vi "Raster_Scan_FSRS.vi"() -> ()   [LabVIEW 2014] (continued)
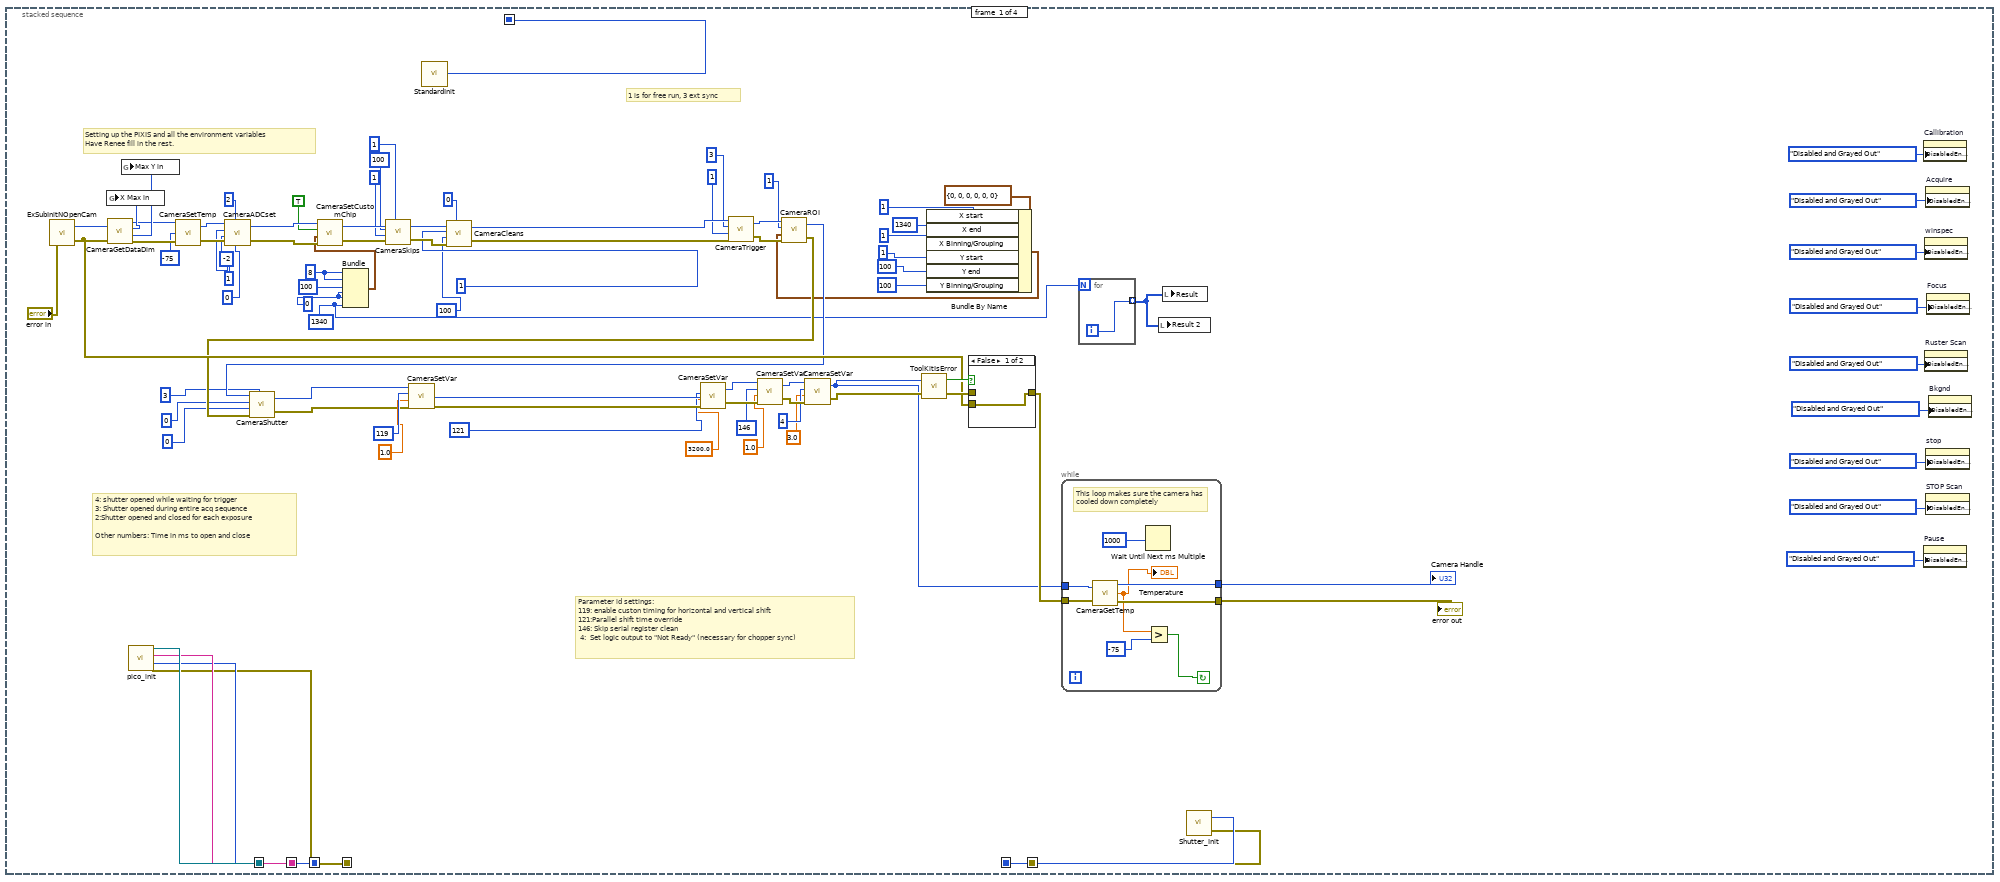
[diagram p2: hidden frame]
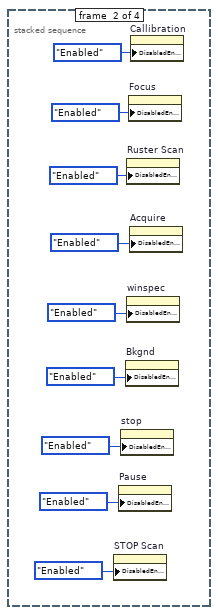
[diagram p4: hidden frame]
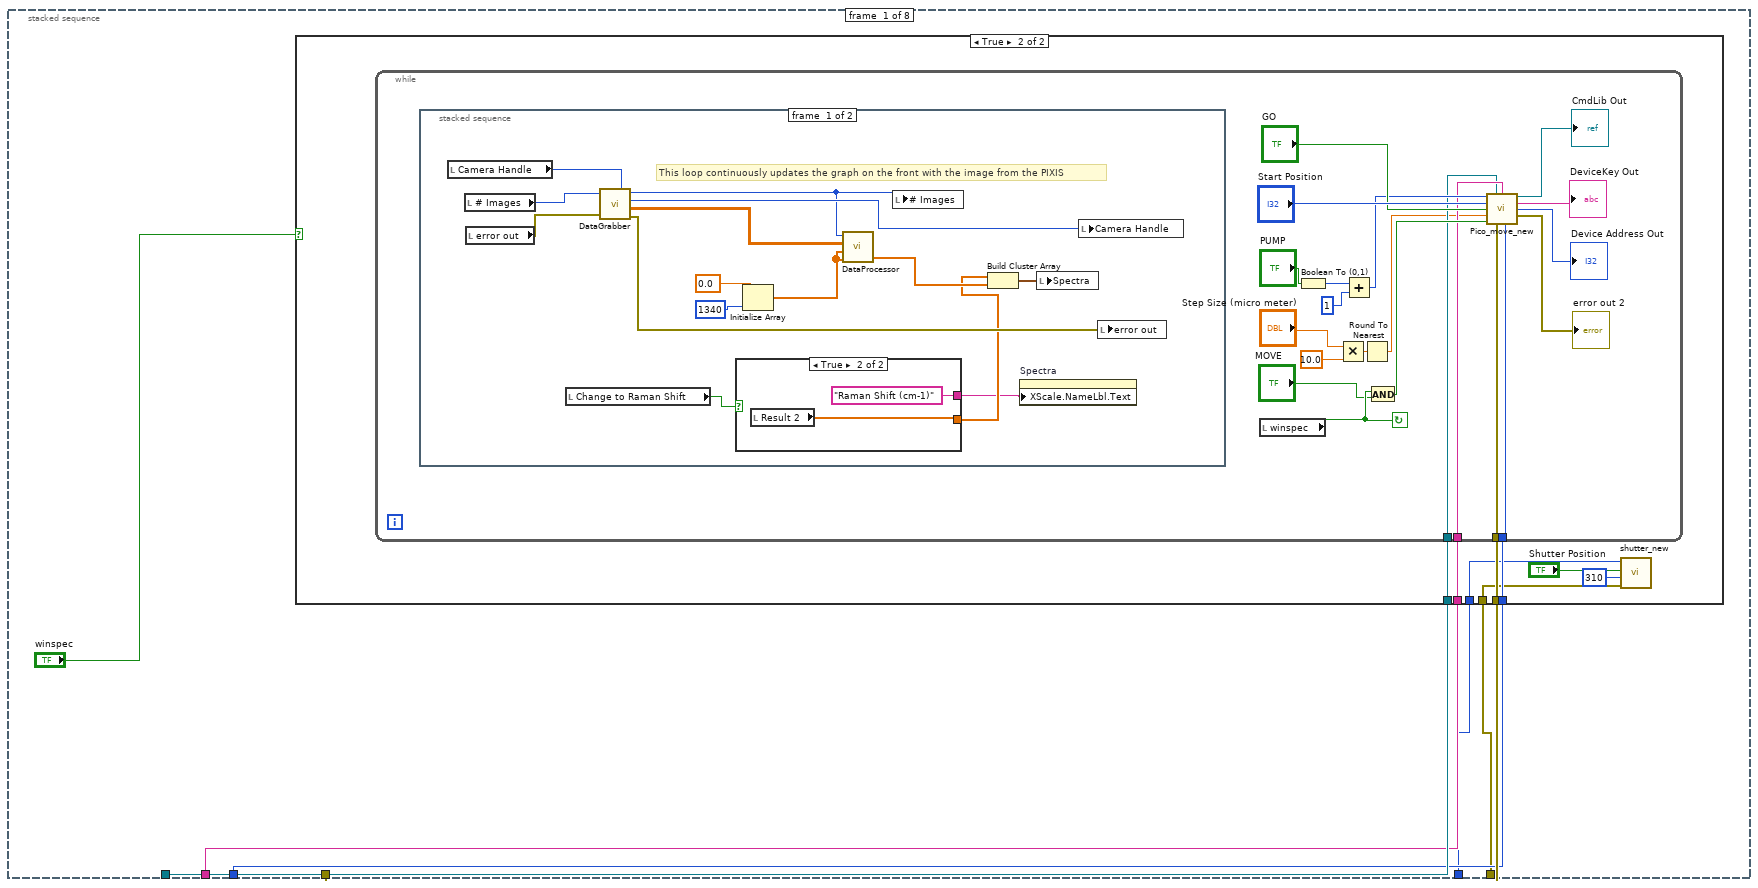
[diagram p5: hidden frame]
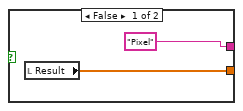
[diagram p7: hidden frame]
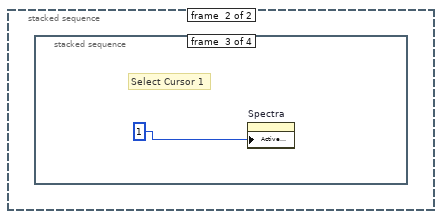
[diagram p8: hidden frame]
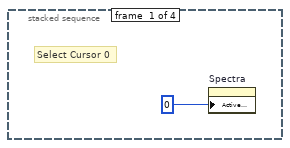
[diagram p9: hidden frame]
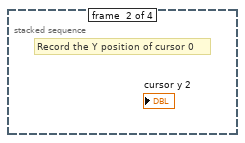
[diagram p10: hidden frame]
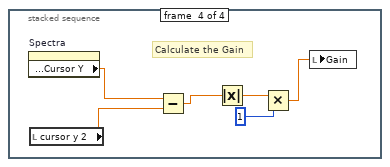
[diagram p11: hidden frame]
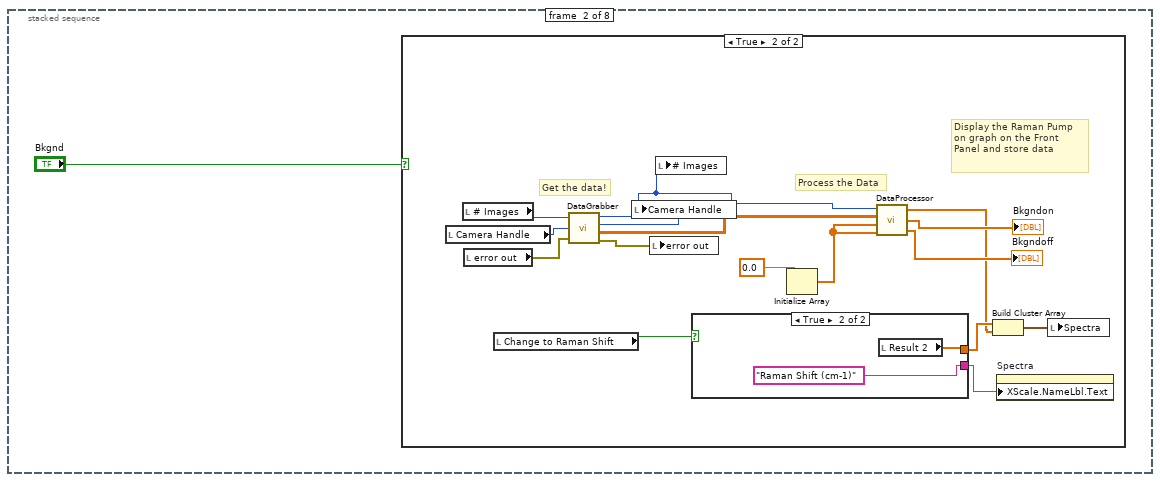
[diagram p12: hidden frame]
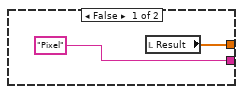
[diagram p14: hidden frame]
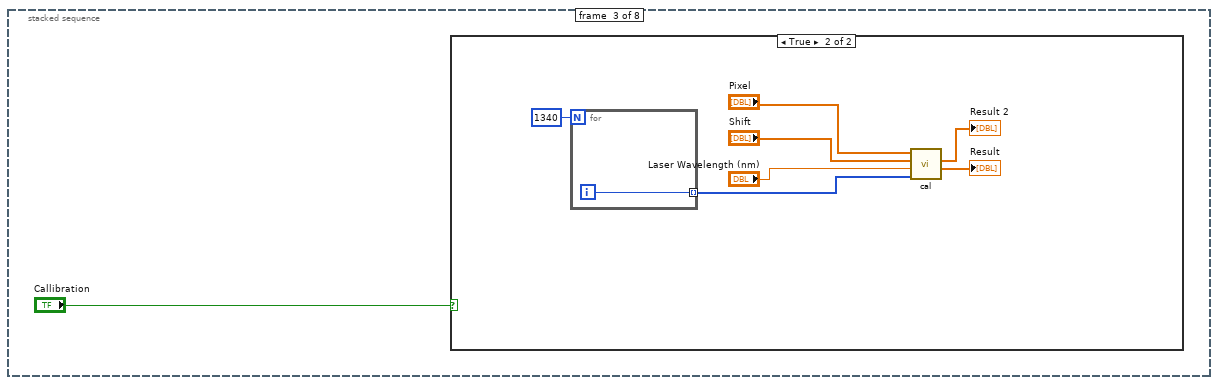
[diagram p15: hidden frame]
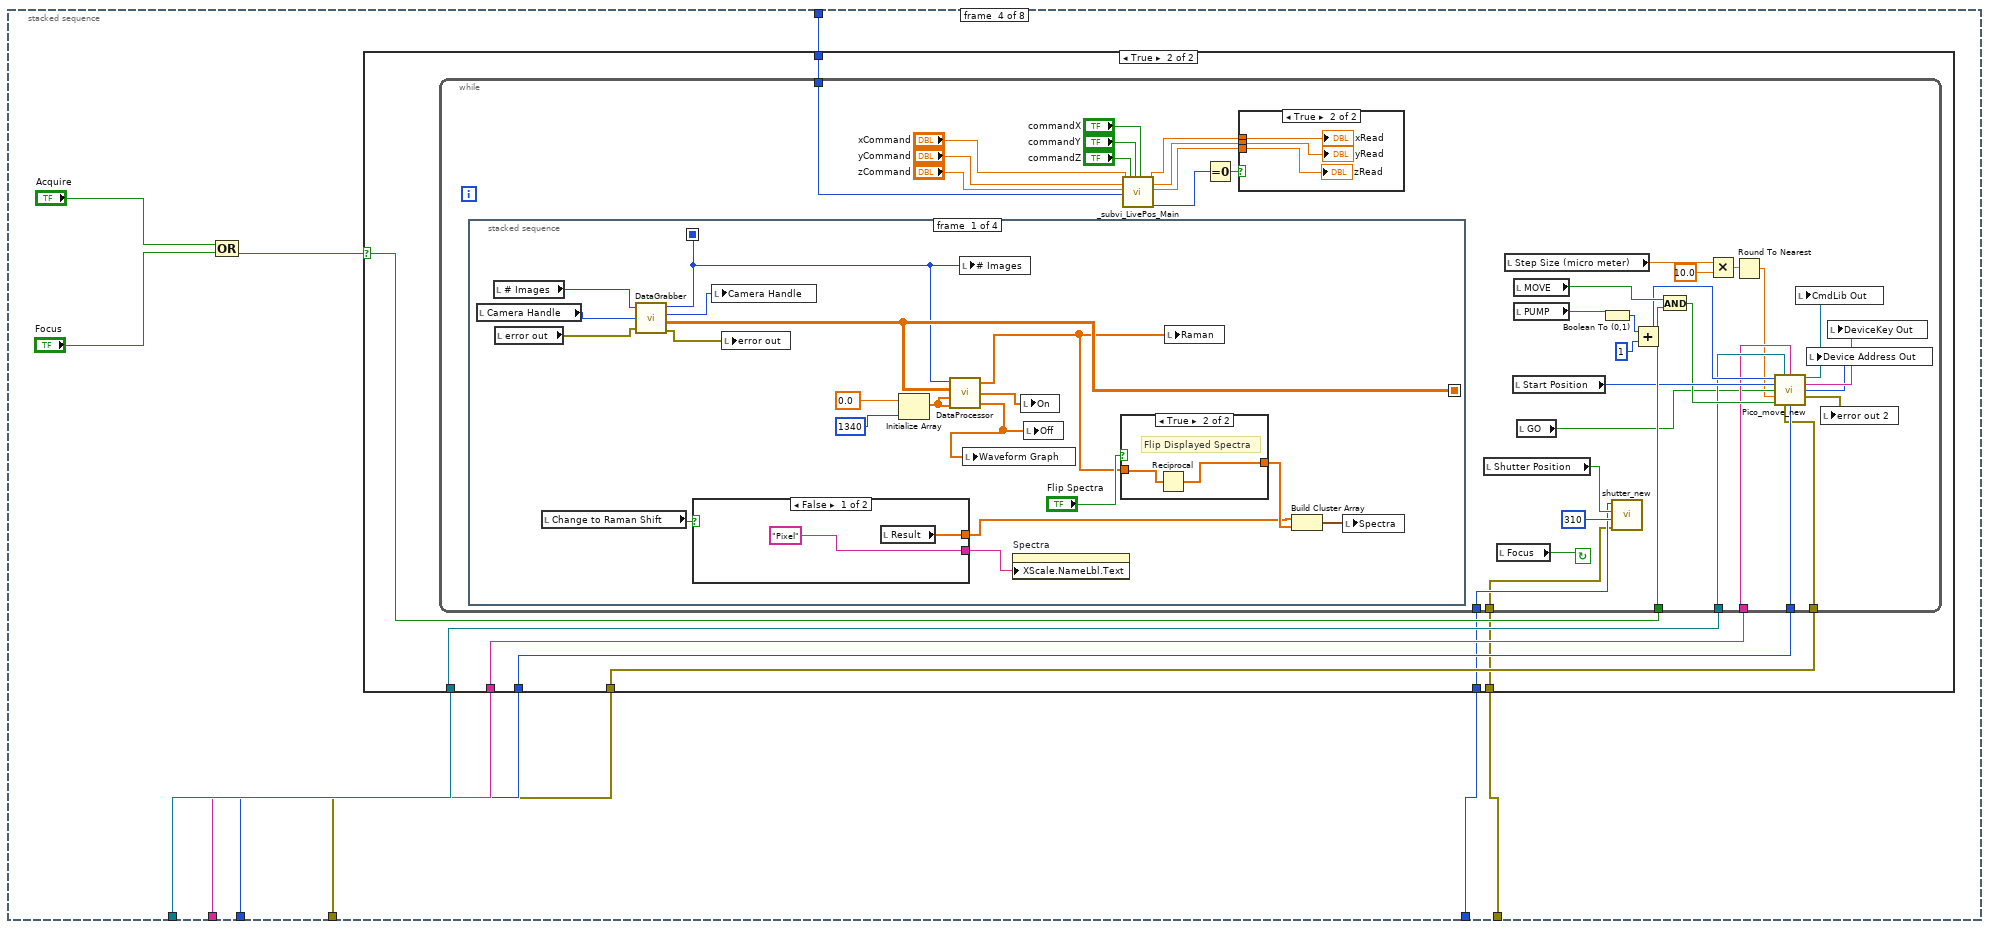
[diagram p17: hidden frame]
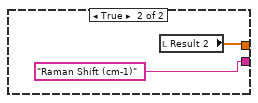
[diagram p20: hidden frame]
                      n390 = Array Size(array="Timepoints") -> (size(s)=w773:i32)
                      n391 = for {
                        N: w773 -> [_]
                        tunnel: "Timepoints" -> [w776]
                        tunnel: w770 -> [w775]
                        tunnel: w771 -> [_]
                        tunnel: w770 -> [_]
                        i -> [w774]
                        n392 = stacked-sequence {
                          seq-local: [_ _ _ w847 _ _ _ _ _ _] -> [_ _ _ _ _ w863 _ _ _ _]
                          seq-local: [_ _ _ w845 _ _ _ _ _ _] -> [_ _ _ _ _ w860 _ _ _ _]
                          tunnel: w774 -> [w778 w828 _ _ _ _ w872 _ _ _]
                          tunnel: w776 -> [_ w829 _ _ _ _ w871 _ _ _]
                          tunnel: w775 -> [w780 _ _ _ _ _ w869 _ _ _]
                          frame #0 {
                            n393 = local read "GndNum"() -> (w779:u32)
                            n394 = Quotient & Remainder(x=w778, y=w779) -> (x-y*floor(x/y)=w782:u32, floor(x/y)=w777:u32)
                            n395 = Equal To 0?(x=w782) -> (x = 0?=w781:bool)
                            n396 = case shown="True" w781 {
                              tunnel: w780 -> [_ w784]
                              tunnel: w777 -> [_ w783]
                              frame False {
                              }
                              frame True {
                                # "Here we take a ground spectrum"
                                n397 = stacked-sequence {
                                seq-local: [w795 _] -> [_ _]
                                tunnel: w784 -> [_ w818]
                                tunnel: w783 -> [_ w808]
                                frame #0 {
                                n398 = local read "Camera Handle 2"() -> (w801:u32)
                                n399 = local read "# Images 2"() -> (w795:u16)
                                n400 = local read "error out 3"() -> (w800:errorcluster)
                                n401 = call "DataGrabber.vi"("# Images In"=w795, "Camera Handle"=w801, "error in (no error)"=w800) -> ("# Images Out"=w790:u16, "Camera Handle"=w798:u32, "Data"=w796:dbl[][], "error out"=w799:errorcluster)
                                n402 = local write "Camera Handle 2"(w798) -> ()
                                n403 = local write "error out 3"(w799) -> ()
                                n404 = local write "# Images 2"(w790) -> ()
                                n405 = local read "Change to Raman Shift 2"() -> (w786:bool)
                                n406 = local read "Bkgndoff 2"() -> (w793:dbl[])
                                n407 = local read "Bkgndon 2"() -> (w794:dbl[])
                                n408 = local read "Flip Spectra 2"() -> (w797:bool)
                                n409 = call "DataProcessor.vi"("PumpOffBkgd"=w793, "PumpOnBkgd"=w794, "Data"=w796, "# of Images"=w790) -> ("PumpOff"=w785:dbl[], "PumpOn"=w791:dbl[], "Raman"=w792:dbl[])
                                "Ground 2" <- w792
                                n410 = local write "Wave"(w785) -> ()
                                n411 = local write "On"(w791) -> ()
                                n412 = local write "Off"(w785) -> ()
                                n413 = case shown="False" w786 {
                                tunnel: [w802 w803] -> w787
                                frame False {
                                n414 = local read "Result 4"() -> (w802:dbl[])
                                }
                                frame True {
                                n415 = local read "Result 3"() -> (w803:dbl[])
                                }
                                }
                                n416 = case shown="True" w797 {
                                tunnel: w792 -> [w804 w806]
                                tunnel: [w804 w805] -> w789
                                frame False {
                                }
                                frame True {
                                n417 = Reciprocal(x=w806) -> (1/x=w805:dbl[])
                                }
                                }
                                n418 = Build Cluster Array(w787, w789) -> (w788:cluster{dbl, dbl}[])
                                n419 = local write "Spectra"(w788) -> ()
                                }
                                frame #1 {
                                # "Here we save the ground spectrum"
                                n420 = local read "Filename 2"() -> (w820:string)
                                n421 = local read "Path 2"() -> (w822:string)
                                n422 = Format Into String(w818) -> (resulting string=w817:string)  [unwired: 3 in, 1 out]
                                n423 = Format Into String(w808) -> (resulting string=w810:string)  [unwired: 3 in, 1 out]
                                n424 = Concatenate Strings(w822, "\\", w820, "_", w817, "_", w810, "gr") -> (w816:string)
                                n425 = local read "Ground"() -> (w807:dbl[])
                                n426 = local read "On"() -> (w824:dbl[])
                                n427 = local read "Off"() -> (w823:dbl[])
                                n428 = String To Path(string=w816) -> (path=w812:path)
                                n429 = Build Array(w807, w824, w823) -> (w813:dbl[][])
                                n430 = call-poly <vilib>:"Write To Spreadsheet File.vi"("transpose? (no:F)"=TRUE, "format (%.3f)"="%.7f", "2D data"=w813, "file path (dialog if empty)"=w812) -> ()  [unwired: 4 in, 1 out]
                                }
                                }
                              }
                            }
                          }
                          frame #1 {
                            n431 = Index Array(array=w829, index=w828) -> (element=w827:dbl)
                            n432 = local read "t=0 Position"() -> (w831:dbl)
                            n433 = Multiply(x=w827, y=0.00015) -> (x*y=w834:dbl)
                            n434 = Add(x=w834, y=w831) -> (x+y=w826:dbl)
                            n435 = Absolute Value(x=w826) -> (abs(x)=w833:dbl)
                            n436 = Less?(x=w833, y=49.9) -> (x < y?=w825:bool)
                            n437 = case shown="True" w825 {
                              tunnel: w826 -> [_ w838]
                              frame False {
                              }
                              frame True {
                                n438 = local read "PI Stage Error"() -> (w837:errorcluster)
                                n439 = call "pi_scan.vi"("error in"=w837, "Start Position"=w838) -> ("error out"=w836:errorcluster, "element"=w835:dbl)  [unwired: 8 in]
                                n440 = Build Array(w835) -> (w839:dbl[])
                                n441 = local write "PI Stage Error"(w836) -> ()
                                n442 = local write "Position"(w839) -> ()
                              }
                            }
                          }
                          frame #2 {
                            # "Open Actinic Pump shutter"
                            n443 = call "shutter.vi"("error in"="shutter error in", "Shutter Position"=TRUE) -> ("error out"=→"shutter error out":errorcluster, "Status"=→"Shutter status":string)  [unwired: 1 in]
                            n444 = Wait (ms)(milliseconds to wait=50) -> ()  [unwired: 1 out]
                          }
                          frame #3 {
                            # "Here we take the data for the given time point"
                            n445 = local read "Camera Handle 2"() -> (w850:u32)
                            n446 = local read "error out 3"() -> (w851:errorcluster)
                            n447 = call "DataGrabber.vi"("# Images In"="# Images 2", "Camera Handle"=w850, "error in (no error)"=w851) -> ("# Images Out"=w845:u16, "Camera Handle"=w848:u32, "Data"=w847:dbl[][], "error out"=w846:errorcluster)
                            n448 = local write "Camera Handle 2"(w848) -> ()
                            n449 = local write "error out 3"(w846) -> ()
                            n450 = local write "# Images 2"(w845) -> ()
                          }
                          frame #4 {
                            # "Actinic Pump Shutter Close"
                            n451 = local read "shutter error in"() -> (w855:errorcluster)
                            n452 = call "shutter.vi"("error in"=w855, "Shutter Position"=FALSE) -> ("error out"=w853:errorcluster, "Status"=w854:string)  [unwired: 1 in]
                            n453 = local write "shutter error out"(w853) -> ()
                            n454 = local write "Shutter status"(w854) -> ()
                            n455 = Wait (ms)(milliseconds to wait=50) -> ()  [unwired: 1 out]
                          }
                          frame #5 {
                            n456 = local read "Bkgndon 2"() -> (w862:dbl[])
                            n457 = local read "Bkgndoff 2"() -> (w861:dbl[])
                            n458 = call "DataProcessor.vi"("PumpOffBkgd"=w861, "PumpOnBkgd"=w862, "Data"=w863, "# of Images"=w860) -> ("PumpOff"=w857:dbl[], "PumpOn"=→"On 2":dbl[], "Raman"=→"Raman 2":dbl[])
                            n459 = local write "Wave"(w857) -> ()
                          }
                          frame #6 {
                            n460 = Index Array(array=w871, index=w872) -> (element=w870:dbl)
                            n461 = call "tppathcr.vi"("input"=w870) -> ("out"=w873:string)
                            n462 = Format Into String(w869) -> (resulting string=w868:string)  [unwired: 3 in, 1 out]
                            n463 = Concatenate Strings("Path 2", "\\", "Filename 2", "_", w873, "exc", w868) -> (w879:string)
                            n464 = local read "Raman 2"() -> (w864:dbl[])
                            n465 = local read "On 2"() -> (w867:dbl[])
                            n466 = local read "Off"() -> (w866:dbl[])
                            n467 = String To Path(string=w879) -> (path=w875:path)
                            n468 = Build Array(w864, w867, w866) -> (w880:dbl[][])
                            n469 = call-poly <vilib>:"Write To Spreadsheet File.vi"("transpose? (no:F)"=TRUE, "format (%.3f)"="%.7f", "2D data"=w880, "file path (dialog if empty)"=w875) -> ()  [unwired: 4 in, 1 out]
                          }
                          frame #7 {
                            n470 = case shown="True" "ShowRaw" {
                              frame False {
                                n471 = local read "Flip Spectra 2"() -> (w892:bool)
                                n472 = local read "Ground 2"() -> (w890:dbl[])
                                n473 = local read "Raman 2"() -> (w891:dbl[])
                                n474 = local read "Change to Raman Shift 2"() -> (w884:bool)
                                n475 = case shown="True" w892 {
                                tunnel: w891 -> [w896 w900]
                                tunnel: [w896 w899] -> w889
                                tunnel: w890 -> [w895 w898]
                                tunnel: [w895 w897] -> w888
                                frame False {
                                }
                                frame True {
                                n476 = Reciprocal(x=w898) -> (1/x=w897:dbl[])
                                n477 = Reciprocal(x=w900) -> (1/x=w899:dbl[])
                                }
                                }
                                n478 = case shown="True" w884 {
                                tunnel: [w893 w894] -> w885
                                frame False {
                                n479 = local read "Result 3"() -> (w893:dbl[])
                                }
                                frame True {
                                n480 = local read "Result 4"() -> (w894:dbl[])
                                }
                                }
                                n481 = Subtract(x=w889, y=w888) -> (x-y=w887:dbl[])
                                n482 = Build Cluster Array(w885, w887) -> (w886:cluster{dbl, "Numeric":dbl}[])
                                n483 = local write "Spectra"(w886) -> ()
                              }
                              frame True {
                                n484 = local read "Flip Spectra 2"() -> (w905:bool)
                                n485 = local read "Change to Raman Shift 2"() -> (w902:bool)
                                n486 = local read "Raman 2"() -> (w906:dbl[])
                                n487 = case shown="False" w905 {
                                tunnel: w906 -> [w909 w911]
                                tunnel: [w909 w910] -> w904
                                frame False {
                                }
                                frame True {
                                n488 = Reciprocal(x=w911) -> (1/x=w910:dbl[])
                                }
                                }
                                n489 = case shown="True" w902 {
                                tunnel: [w907 w908] -> w903
                                frame False {
                                n490 = local read "Result 3"() -> (w907:dbl[])
                                }
                                frame True {
                                n491 = local read "Result 4"() -> (w908:dbl[])
                                }
                                }
                                n492 = Build Cluster Array(w903, w904) -> (w901:cluster{dbl, "Numeric":dbl}[])
                                n493 = local write "Spectra"(w901) -> ()
                              }
                            }
                          }
                          frame #8 {
                            n494 = stacked-sequence {
                              frame #0 {
                                n495 = property on="Spectra" class="XYGraph (strict)"("Active Cursor"=0) -> ()  [unwired: 2 in, 2 out]
                              }
                              frame #1 {
                                n496 = property on="Spectra" class="XYGraph (strict)"() -> ("Cursor.Cursor Position:Cursor Y"=w914:dbl)  [unwired: 2 in, 2 out]
                                n497 = local read "Change to Raman Shift 2"() -> (w915:bool)
                                n498 = local write "cursor y"(w914) -> ()
                                n499 = case shown="False" w915 {
                                tunnel: ["Pixel" ("X Scale.Name Label.Text") "Raman Shift (cm-1)" ("X Scale.Name Label.Text")] -> w913
                                frame False {
                                }
                                frame True {
                                }
                                }
                                n500 = property on="Spectra" class="XYGraph (strict)"("XScale.NameLbl.Text"=w913) -> ()  [unwired: 2 in, 2 out]
                              }
                              frame #2 {
                                n501 = property on="Spectra" class="XYGraph (strict)"("Active Cursor"=1) -> ()  [unwired: 2 in, 2 out]
                              }
                              frame #3 {
                                n502 = property on="Spectra" class="XYGraph (strict)"() -> ("Cursor.Cursor Position:Cursor Y"=w919:dbl)  [unwired: 2 in, 2 out]
                                n503 = local read "cursor y"() -> (w920:dbl)
                                n504 = Subtract(x=w919, y=w920) -> (x-y=w922:dbl)
                                n505 = Absolute Value(x=w922) -> (abs(x)=w924:dbl)
                                n506 = Multiply(x=w924, y=100) -> (x*y=w921:dbl)
                                n507 = local write "Gain 2"(w921) -> ()
                              }
                            }
                          }
                          frame #9 {
                            n508 = while {
                              stop <- "Pause 2" continue-if-true
                            }
                          }
                        }
                      }
                    }
                  }
                }
              }
            }
          }
          frame #6 {
            n509 = case shown="True" "Save" {
              frame False {
              }
              frame True {
                n510 = local read "Raman"() -> (w949:dbl[])
                n511 = local read "Off"() -> (w947:dbl[])
                n512 = local read "On"() -> (w948:dbl[])
                n513 = local read "Path"() -> (w946:string)
                n514 = Build Array(w949, w948, w947) -> (w940:dbl[][])
                n515 = local read "Filename"() -> (w944:string)
                n516 = Concatenate Strings(w946, "\\", w944) -> (w943:string)
                n517 = String To Path(string=w943) -> (path=w939:path)
                n518 = call-poly <vilib>:"Write To Spreadsheet File.vi"("transpose? (no:F)"=TRUE, "format (%.3f)"="%.7f", "2D data"=w940, "file path (dialog if empty)"=w939) -> ()  [unwired: 4 in, 1 out]
              }
            }
            n519 = case shown="True" "subtract" {
              frame False {
              }
              frame True {
                n520 = local read "Change to Raman Shift"() -> (w957:bool)
                n521 = local read "Subtrarray"() -> (w961:dbl[])
                n522 = local read "Raman"() -> (w960:dbl[])
                n523 = Multiply(x="Scale factor", y=w961) -> (x*y=w959:dbl[])
                n524 = Subtract(x=w960, y=w959) -> (x-y=w955:dbl[])
                n525 = case shown="True" w957 {
                  tunnel: [w964 w966] -> w956
                  tunnel: ["Pixel" ("X Scale.Name Label.Text") "Raman Shift (cm-1)" ("X Scale.Name Label.Text")] -> w958
                  frame False {
                    n526 = local read "Result"() -> (w964:dbl[])
                  }
                  frame True {
                    n527 = local read "Result 2"() -> (w966:dbl[])
                  }
                }
                n528 = property on="Spectra" class="XYGraph (strict)"("XScale.NameLbl.Text"=w958) -> ()  [unwired: 2 in, 2 out]
                n529 = Build Cluster Array(w956, w955) -> (w954:cluster{dbl, dbl}[])
                n530 = local write "Spectra"(w954) -> ()
              }
            }
            n531 = case shown="True" "ChooseBkgdFile" {
              frame False {
              }
              frame True {
                n532 = call-poly <vilib>:"Read From Spreadsheet File.vi"("transpose (no:F)"=TRUE) -> ("first row"=w968:dbl[], "new file path (Not A Path if cancelled)"=→"Background File":path)  [unwired: 6 in, 3 out]
                n533 = Array Subset(array=w968, index=0, length=1340) -> (→"Subtrarray":dbl[])
              }
            }
            n534 = case shown="True" "SetPath" {
              frame False {
              }
              frame True {
                (unwired) 5
                n535 = File Dialog(11:path "C:/DATA") -> (0:w950:errorcluster, 3:w953:path)  [unwired: 6 in, 2 out]
                n536 = Unbundle(w950) -> ()  [unwired: 3 out]
                n537 = Path To String(path=w953) -> (string=w951:string)
                n538 = local write "Path"(w951) -> ()
              }
            }
            n539 = case shown="True" "Boolean" {
              frame False {
              }
              frame True {
                n540 = local read "Path"() -> (w935:string)
                n541 = local read "Filename"() -> (w937:string)
                n542 = Concatenate Strings(w935, "\\", w937) -> (w938:string)
                n543 = String To Path(string=w938) -> (path=w934:path)
                n544 = local read "Off"() -> (w931:dbl[])
                n545 = call-poly <vilib>:"Write To Spreadsheet File.vi"("transpose? (no:F)"=TRUE, "format (%.3f)"="%.7f", "1D data"=w931, "file path (dialog if empty)"=w934) -> ()  [unwired: 4 in, 1 out]
              }
            }
          }
          frame #7 {
            n546 = case shown="True" "Time" {
              frame False {
              }
              frame True {
                n547 = while {
                  shift-right: [w975] -> _
                  shift-left: _ -> [w974]
                  i -> [w976]
                  stop <- "?" stop-if-true
                  n548 = stacked-sequence {
                    seq-local: [w978 _ _] -> [_ _ w1024]
                    tunnel: w976 -> [_ w1005 _]
                    tunnel: [_ _ w1021] -> w975
                    tunnel: w974 -> [_ _ w1020]
                    frame #0 {
                      n549 = local read "Change to Raman Shift"() -> (w980:bool)
                      n550 = local read "# Images"() -> (w979:u16)
                      n551 = local read "Camera Handle"() -> (w996:u32)
                      n552 = local read "error out"() -> (w995:errorcluster)
                      n553 = call "DataGrabber.vi"("# Images In"=w979, "Camera Handle"=w996, "error in (no error)"=w995) -> ("# Images Out"=w989:u16, "Camera Handle"=w993:u32, "Data"=w992:dbl[][], "error out"=w994:errorcluster)
                      n554 = local write "Camera Handle"(w993) -> ()
                      n555 = local write "error out"(w994) -> ()
                      n556 = case shown="False" w980 {
                        tunnel: [w998 w1000] -> w978
                        tunnel: ["Pixel" ("X Scale.Name Label.Text") "Raman Shift (cm-1)" ("X Scale.Name Label.Text")] -> w982
                        frame False {
                          n557 = local read "Result"() -> (w998:dbl[])
                        }
                        frame True {
                          n558 = local read "Result 2"() -> (w1000:dbl[])
                        }
                      }
                      n559 = local write "# Images"(w989) -> ()
                      n560 = local read "Bkgndoff"() -> (w990:dbl[])
                      n561 = local read "Bkgndoff"() -> (w991:dbl[])
                      n562 = call "DataProcessor.vi"("PumpOffBkgd"=w990, "PumpOnBkgd"=w991, "Data"=w992, "# of Images"=w989) -> ("PumpOff"=w988:dbl[], "PumpOn"=w987:dbl[], "Raman"=w981:dbl[])
                      n563 = local read "Flip Spectra"() -> (w984:bool)
                      n564 = property on="Spectra" class="XYGraph (strict)"("XScale.NameLbl.Text"=w982) -> ()  [unwired: 2 in, 2 out]
                      n565 = local write "On"(w987) -> ()
                      n566 = local write "Off"(w988) -> ()
                      n567 = Not(x=w984) -> (.not. x?=w985:bool)
                      n568 = case shown="True" w985 {
                        tunnel: w981 -> [w1001 w1003]
                        tunnel: [w1002 w1003] -> w986
                        frame False {
                          n569 = Reciprocal(x=w1001) -> (1/x=w1002:dbl[])
                        }
                        frame True {
                        }
                      }
                      n570 = Build Cluster Array(w978, w986) -> (w983:cluster{dbl, dbl}[])
                      n571 = local write "Spectra"(w983) -> ()
                      n572 = local write "Raman"(w981) -> ()
                    }
                    frame #1 {
                      # "Here we save spectrum for each special point"
                      n573 = Increment(x=w1005) -> (x+1=w1004:i32)
                      n574 = local read "Filename"() -> (w1008:string)
                      n575 = local read "Path"() -> (w1010:string)
                      n576 = Format Into String(w1004) -> (resulting string=w1006:string)  [unwired: 3 in, 1 out]
                      n577 = Concatenate Strings(w1010, "\\", w1008, "_", w1006) -> (w1011:string)
                      n578 = local read "Off"() -> (w1018:dbl[])
                      n579 = local read "On"() -> (w1017:dbl[])
                      n580 = local read "Raman"() -> (w1014:dbl[])
                      n581 = String To Path(string=w1011) -> (path=w1015:path)
                      n582 = Build Array(w1014, w1018, w1017) -> (w1016:dbl[][])
                      n583 = local write "File_name"(w1011) -> ()
                      n584 = call-poly <vilib>:"Write To Spreadsheet File.vi"("transpose? (no:F)"=TRUE, "format (%.3f)"="%.7f", "2D data"=w1016, "file path (dialog if empty)"=w1015) -> ()  [unwired: 4 in, 1 out]
                    }
                    frame #2 {
                      # "Peak fitting and intergation"
                      n585 = local read "Raman"() -> (w1025:dbl[])
                      n586 = property on="Spectra" class="XYGraph (strict)"("Active Cursor"=u32 1) -> ("Cursor.Cursor X"=w1027:dbl)  [unwired: 2 in, 2 out]
                      n587 = local read "Enum"() -> (w1022:enum16{"Lorantzian", "fano", "gaussian"})
                      n588 = property on="Spectra" class="XYGraph (strict)"("Active Cursor"=u32 0) -> ("Cursor.Cursor X"=w1028:dbl)  [unwired: 2 in, 2 out]
                      n589 = call "fit_new.vi"("Cursor1 2"=w1027, "Cursor1"=w1028, "array 2"=w1024, "array"=w1025, "Enum"=w1022, "Initial Parameters"="Fano initial Parameters 2") -> ("Intergrate"=w1023:dbl, "Fit"=w1019:dbl)  [unwired: 4 in]
                      n590 = local write "FIT"(w1019) -> ()
                      n591 = local write "AREA"(w1023) -> ()
                      n592 = Build Array (concatenate)(w1020, w1019) -> (w1021:dbl[])
                      "Waveform Graph" <- w1021
                    }
                  }
                }
              }
            }
          }
        }
      }
    }
    frame #3 {
      n593 = local read "DeviceKey Out"() -> (w1033:string)
      n594 = local read "error out 2"() -> (w1032:errorcluster)
      n595 = local read "CmdLib Out"() -> (w1034:refnum<k24>)
      n596 = stacked-sequence {
        frame #0 {
          n597 = local read "Camera Handle"() -> (w1035:u32)
          n598 = local read "error out"() -> (w1036:errorcluster)
          n599 = call <userlib>:"CameraClose.vi"("error in"=w1036, "Camera Handle"=w1035) -> ("error out"=w1038:errorcluster)
          n600 = call <userlib>:"UninitToolkit.vi"("error in"=w1038) -> ("error out"=w1037:errorcluster)
          n601 = local write "error out"(w1037) -> ()
        }
      }
      n602 = call <instrlib>:"DeviceClose.vi"("error in (no error)"=w1032, "DeviceKey In"=w1033, "CmdLib In"=w1034) -> ()  [unwired: 2 in, 3 out]
      n603 = dll-call lib="C:/Program Files/Mad City Labs/NanoDrive/Labview Examples/MADLib.dll" fn="MCL_ReleaseHandle"("handle"=w1031) -> ()  [unwired: 5 in, 2 out]
    }
  }
